vi "Authorization Encode String.vi"(8 "error in (no error)":errorcluster, 9 "Volume Serial Number":string, 10 "Property Name":string, 11 "Decoded String":string) -> (0 "error out":errorcluster, 3 "Encoded String":string)   [LabVIEW 2011]
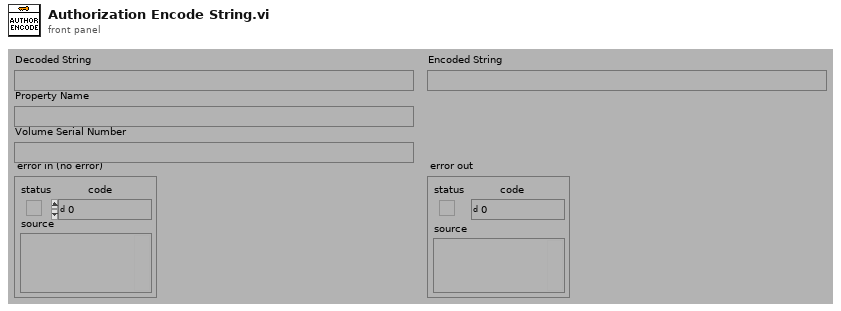
[diagram p1: front panel]
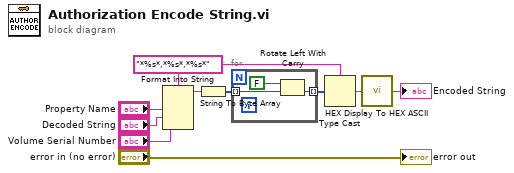
[diagram p0: block diagram]
diagram:
  w6 = "*%s*,*%s*,*%s*" ("format string")
  n1 = Format Into String(format string=w6, "Property Name", "Decoded String", "Volume Serial Number") -> (resulting string=w10:string)  [unwired: 2 in, 1 out]
  n2 = String To Byte Array(string=w10) -> (unsigned byte array=w9:u8[])
  n3 = for {
    tunnel: w9 -> [w13] mode=indexing
    tunnel: [w12] -> w8 mode=indexing
    n4 = Rotate Left With Carry(2:w13, 3:FALSE ("carry")) -> (0:w12:u8)  [unwired: 1 out]
  }
  n5 = Type Cast(type=w6, x=w8) -> (*(type *) &x=w2:string)
  n6 = call "HEX Display To HEX ASCII.vi"("Input ASCII String (HEX Display)"=w2) -> ("Output HEX ASCII (Normal Display)"=→"Encoded String":string)  [unwired: 4 in]
  "error out" <- "error in (no error)"
